vi "make-relative-path.vi"(2 "Relative Path":string="..\\work", 3 "the current VI's path":path) -> (0 "Path as a string":string, 1 "Constructed Path":path)   [LabVIEW 2010]
doc: "для корректной работы требуется подсоединить\nCurrent VI's path из меню\nAll Functions -> File I/O -> File Constants \nтакже, строку для нового пути. Отрабатывается \"..\" - переход в директорию более высокого уровня:\nНапример, вызов из \"D:\\mydir\\tmp\" с параметром \"..\\altdir\" сконструирует путь \"D:\\mydir\\altdir\""
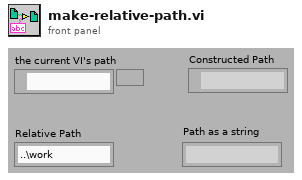
[diagram p1: front panel]
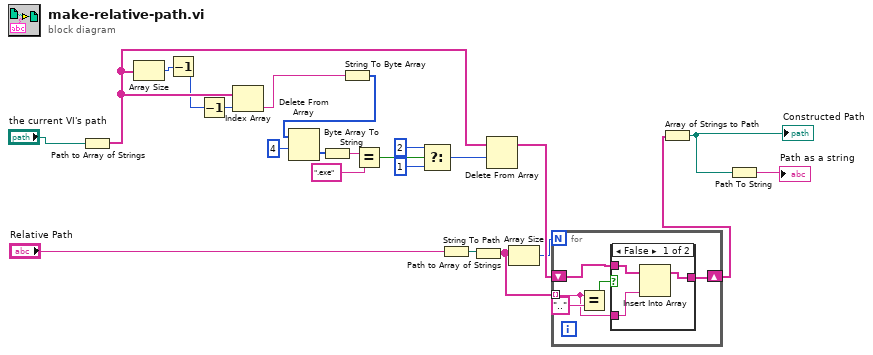
[diagram p0: block diagram]
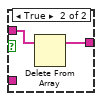
[diagram p2: hidden frame]
diagram:
  n1 = Path to Array of Strings(0:"the current VI's path") -> (2:w17:string[])  [unwired: 1 out]
  n2 = Array Size(array=w17) -> (size(s)=w5:i32)
  n3 = Decrement(x=w5) -> (x-1=w6:i32)
  n4 = Decrement(x=w6) -> (x-1=w7:i32)
  n5 = Index Array(array=w17, index=w7) -> (element=w8:string)
  n6 = String To Byte Array(string=w8) -> (unsigned byte array=w10:u8[])
  n7 = Delete From Array(array=w10, length=4) -> (deleted portion=w11:u8[])  [unwired: 1 in, 1 out]
  n8 = Byte Array To String(unsigned byte array=w11) -> (string=w12:string)
  n9 = Equal?(x=w12, y=".exe") -> (x = y?=w1:bool)
  n10 = Select(t=u16 2, s=w1, f=u16 1) -> (s? t:f=w16:u16)
  n11 = String To Path(string="Relative Path") -> (path=w18:path)
  n12 = Path to Array of Strings(0:w18) -> (2:w21:string[])  [unwired: 1 out]
  n13 = Delete From Array(array=w17, length=w16) -> (array with subset deleted=w22:string[])  [unwired: 1 in, 1 out]
  n14 = Array Size(array=w21) -> (size(s)=w19:i32)
  n15 = for {
    N: w19 -> [_]
    tunnel: w21 -> [w24] mode=indexing
    shift-right: [w25] -> w23
    shift-left: w22 -> [w26]
    n16 = Equal?(x=w24, y="..") -> (x = y?=w27:bool)
    n17 = case shown="False" w27 {
      tunnel: w26 -> [w31 w33]
      tunnel: [w30 w32] -> w25
      tunnel: w24 -> [w29 _]
      frame False {
        n18 = Insert Into Array(array=w31, new element=w29) -> (w30:string[])  [unwired: 1 in]
      }
      frame True {
        n19 = Delete From Array(array=w33) -> (array with subset deleted=w32:string[])  [unwired: 2 in, 1 out]
      }
    }
  }
  n20 = Array of Strings to Path(0:w23) -> (2:w4:path)  [unwired: 1 in]
  "Constructed Path" <- w4
  n21 = Path To String(path=w4) -> (string=→"Path as a string":string)
